vi "Main Process Case.vi"(8 "error in (no error)":errorcluster, 10 "CurrentAction":string, 11 "Main Process Class in":refnum<class "MPC_VirbVision.lvclass">) -> (0 "error out":errorcluster, 1 "KeepCase":bool, 3 "Main Process Class out":refnum<class "MPC_VirbVision.lvclass">)   [LabVIEW 2019, in "MPC_VirbVision.lvclass"]
uses:
  MPC_VirbVision.lvclass
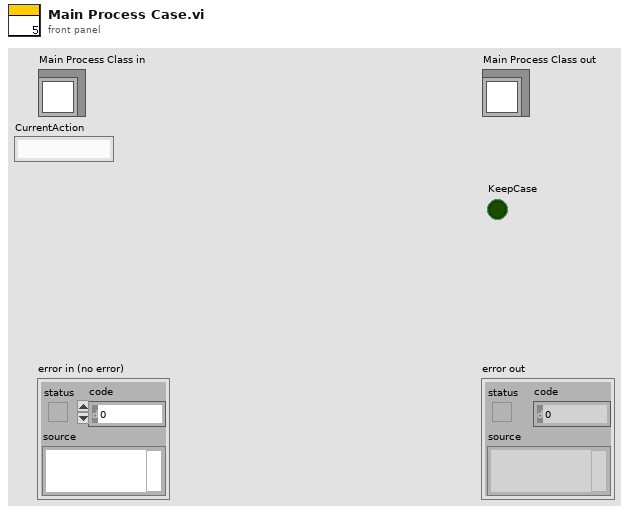
[diagram p1: front panel]
types:
  T1 = cluster{"AutoRunFlg":refnum<vi>, "Action Finish Flg":refnum<vi>, "Remaining Action":refnum<vi>, "Btn_AutoRun":refnum<vi>, "Manual Flg":refnum<vi>, "Sub Process Error":refnum<vi>}
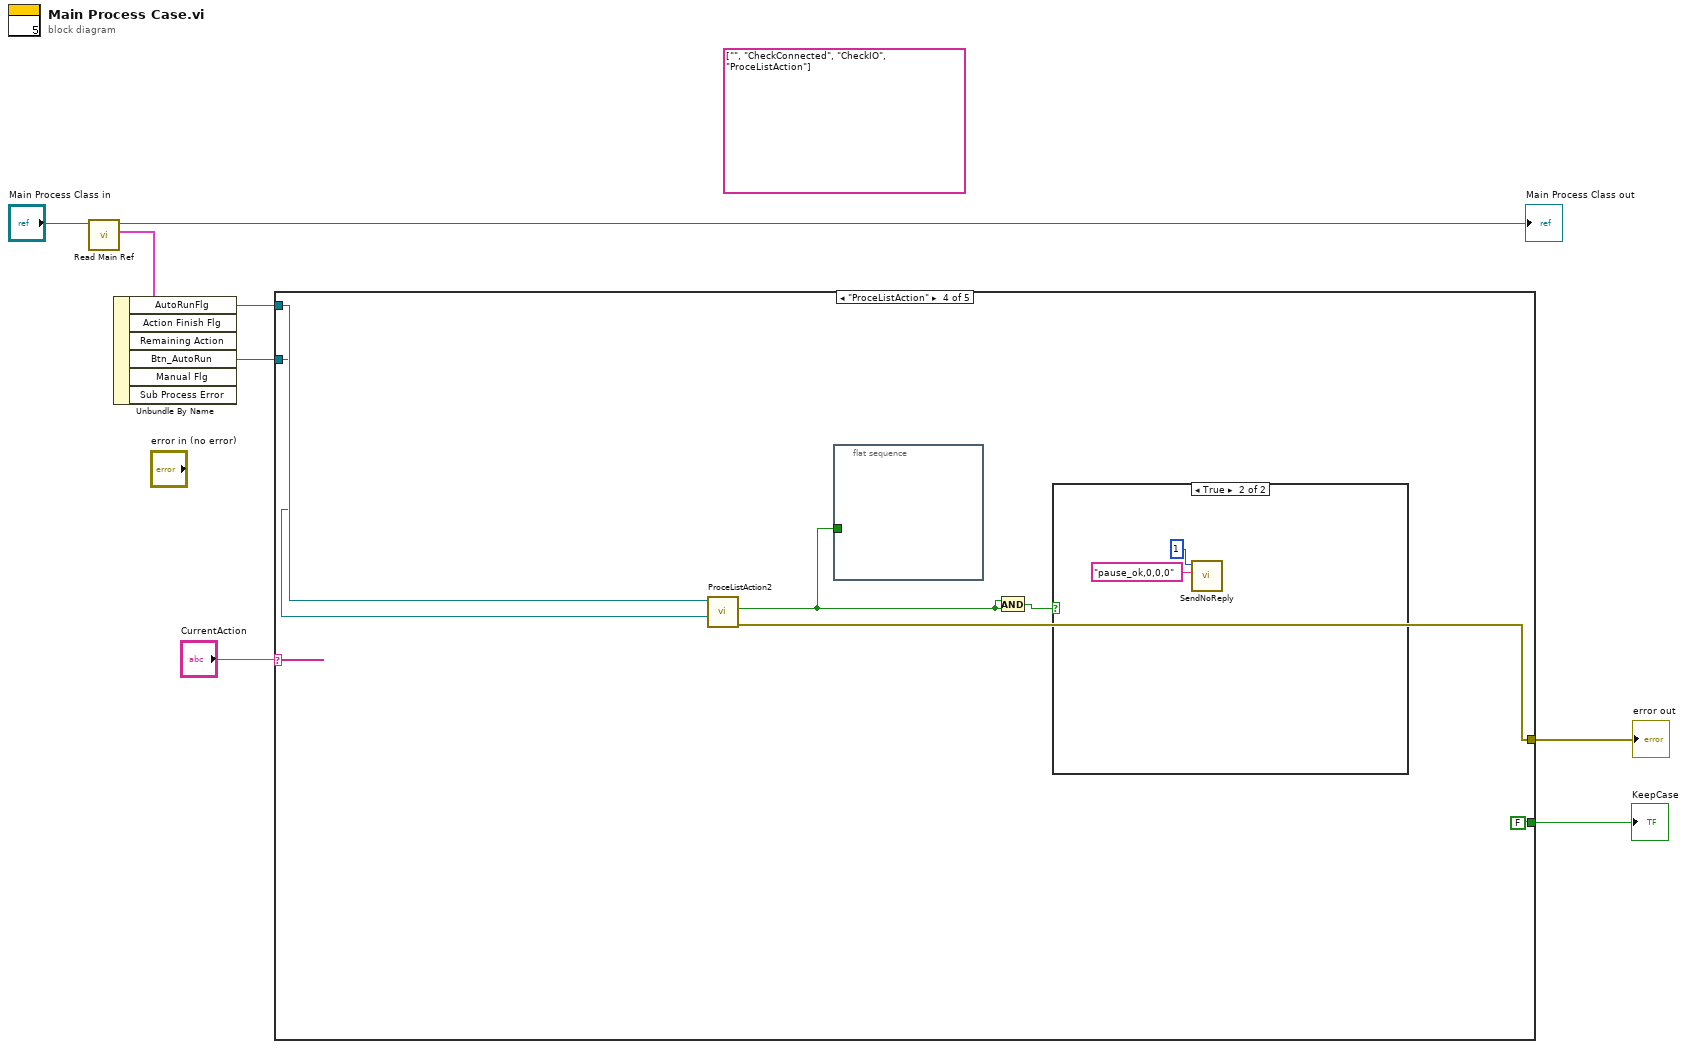
[diagram p0: block diagram]
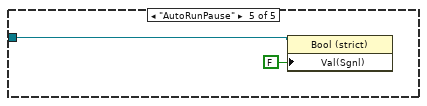
[diagram p6: hidden frame]
diagram:
  (unwired) string[] ["", "CheckConnected", "CheckIO", "ProceListAction"]
  n1 = call-dynamic "Read Main Ref.vi"("Main Process Class in"="Main Process Class in") -> ("Main Ref"=w3:T1, "Main Process Class out"=→"Main Process Class out":refnum<class "MPC_VirbVision.lvclass">)  [unwired: 8 in, 1 out]
  n2 = Unbundle By Name(w3) -> ("AutoRunFlg"=w1:refnum<vi>, "Btn_AutoRun"=w2:refnum<vi>)  [unwired: 4 out]
  n3 = case shown="\"ProceListAction\"" "CurrentAction" {
    tunnel: [_ _ _ w14 _] -> w7
    tunnel: [_ _ _ FALSE _] -> w6
    tunnel: w2 -> [_ _ _ w11 w18]
    tunnel: w1 -> [_ _ _ w12 _]
    frame "False", Default {
    }
    frame "CheckConnected" {
    }
    frame "CheckIO" {
    }
    frame "ProceListAction" {
      n4 = call "ProceListAction2.vi"("Btn_AutoRun"=w11, "AutoRunFlg"=w12) -> ("error out"=w14:errorcluster, "pause"=w9:bool)  [unwired: 8 in]
      n5 = flat-sequence {
        tunnel: w9 -> [_]
        frame #0 {
        }
      }
      n6 = And(x=w9, y=w9) -> (x .and. y?=w10:bool)
      n7 = case shown="True" w10 {
        frame False {
        }
        frame True {
          n8 = call "SendNoReply.vi"("DataIn"="pause_ok,0,0,0", "index"=1) -> ()  [unwired: 9 in, 1 out]
        }
      }
    }
    frame "AutoRunPause" {
      n9 = property class="Bool (strict)"(reference=w18, "Val(Sgnl)"=FALSE ("Value (Signaling)")) -> ()  [unwired: 1 in, 2 out]
    }
  }
  "error out" <- w7
  "KeepCase" <- w6
